vi "test data analysis.vi"() -> ()   [LabVIEW 2013]
uses:
  <vilib>/Utility/file.llb/Read From Spreadsheet File (string).vi
panel:
  out "Pick up Balance  2":cluster{dbl[], dbl[]}(graph)
  in  "탭 컨트롤":enum32{"페이지 1", "페이지 2"}(tab)
  out "Bonding Balance":cluster{dbl[], dbl[]}(graph)
  out "Pick up Balance":cluster{dbl[], dbl[]}(graph)
  out "숫자형":i32
  out "Balance all":cluster{dbl[], dbl[]}(graph)
  in  "balance y":i32
  in  "balance x":i32
  in  "time index 2":i32
  out "temp 그래프 4":dbl[](graph)
  out "temp 그래프 3":dbl[](graph)
  in  "vacuum index":i32
  out "temp 그래프 2":dbl[](graph)
  in  "temp index":i32
  in  "force index":i32
  out "웨이브폼 그래프":dbl[](graph)
  in  "file path":path caption="Data file path"
  out "Data Table":string[][](table)
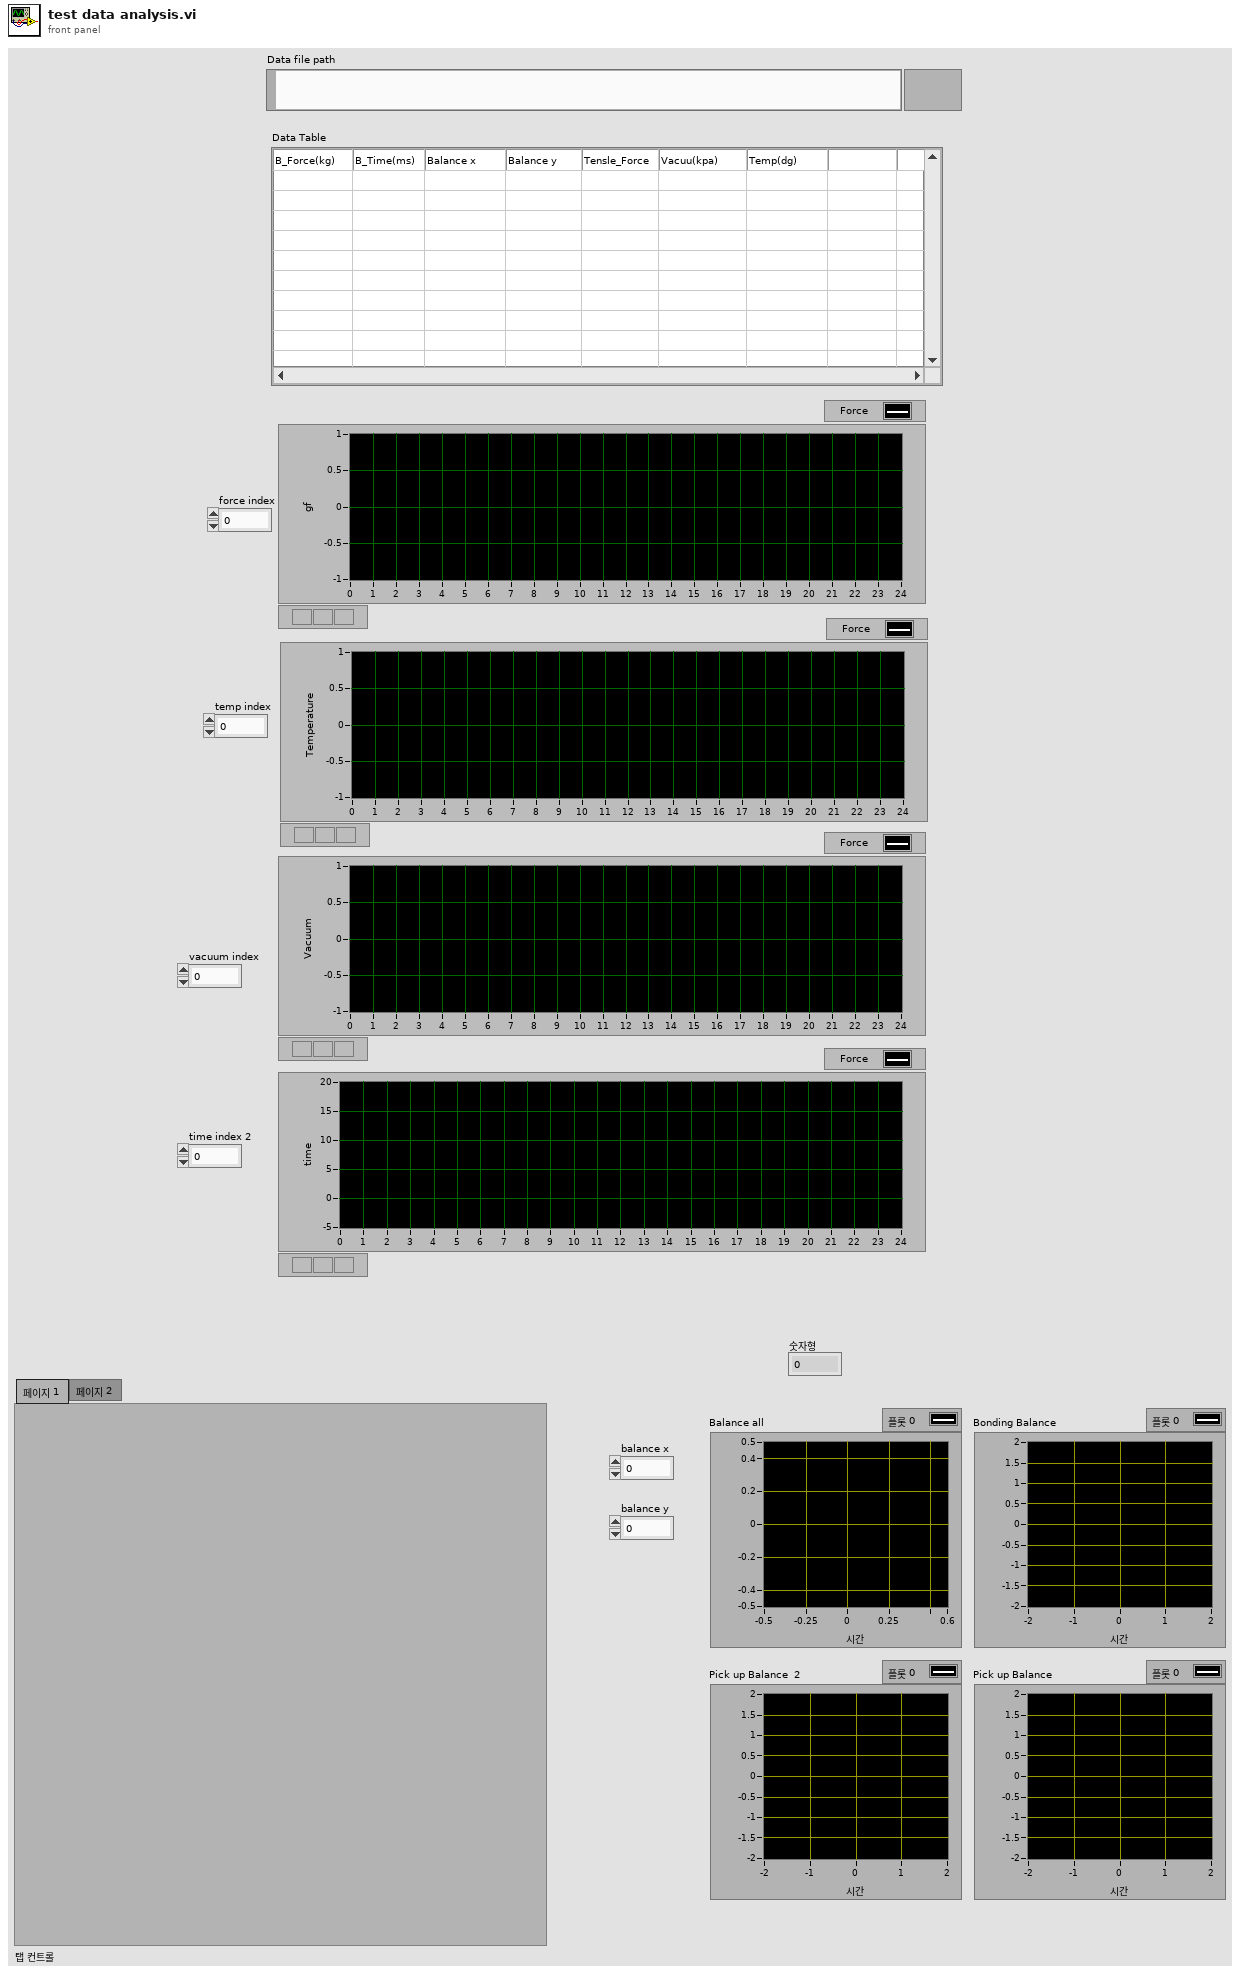
[diagram p1: front panel]
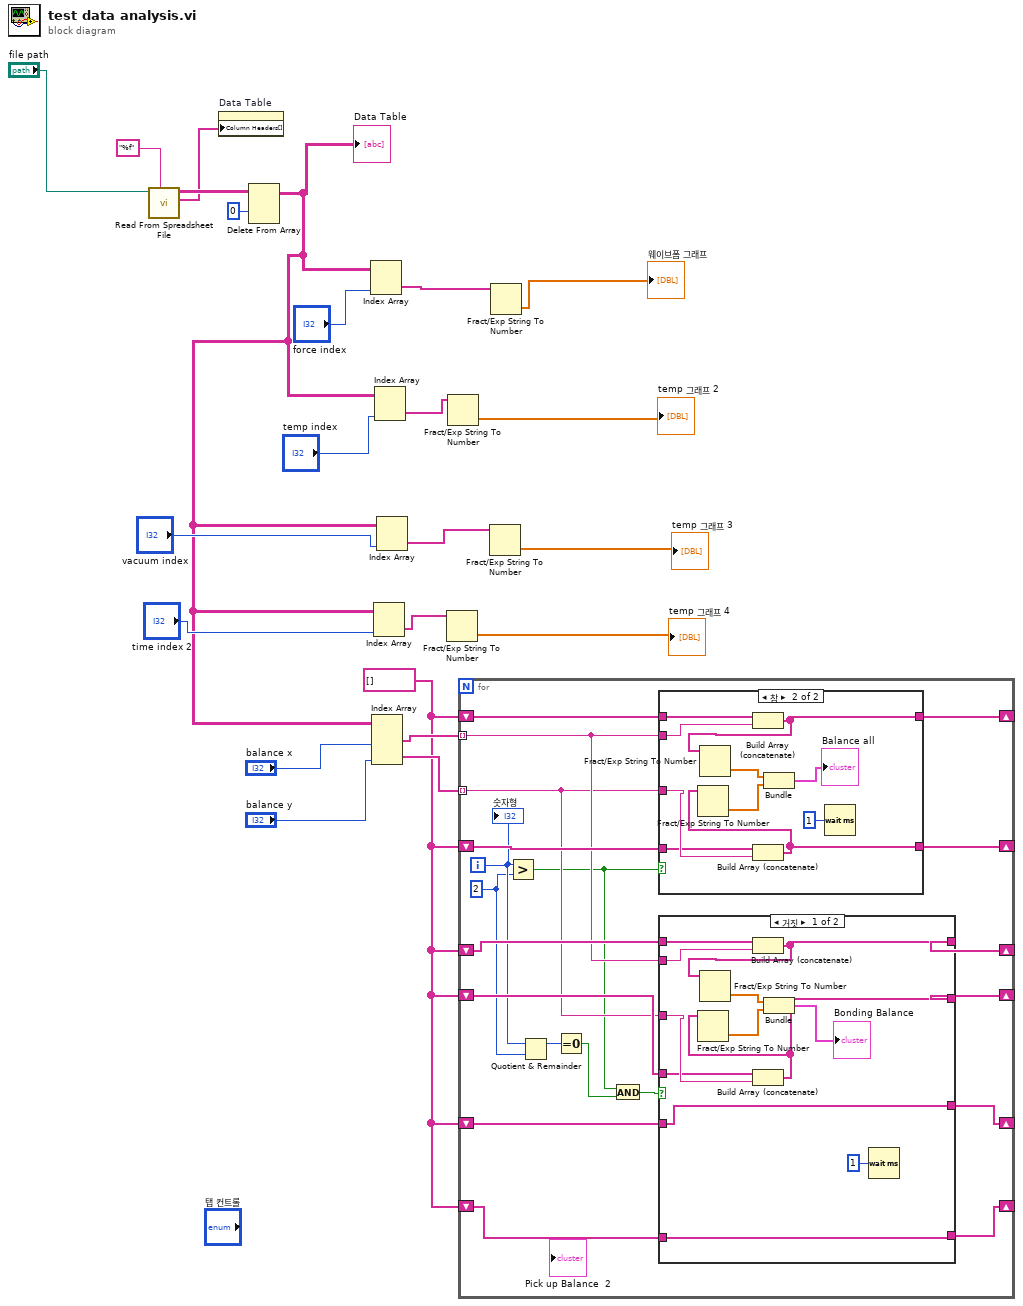
[diagram p0: block diagram]
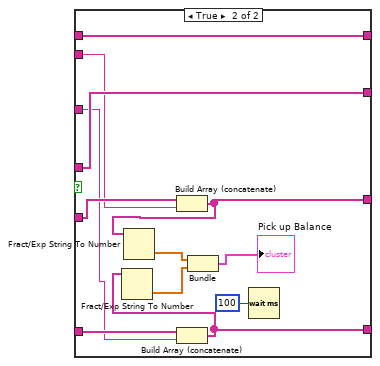
[diagram p2: hidden frame]
diagram:
  w1 = string[] []
  n1 = call-poly <vilib>:"Read From Spreadsheet File.vi"("format (%s)"="%f", "file path (dialog if empty)"="file path") -> ("first row"=w20:string[], "all rows"=w22:string[][])  [unwired: 5 in, 3 out]
  n2 = property on="Data Table" class="Tbl (엄격한)"("Column Headers[]"=w20) -> ()  [unwired: 2 in, 2 out]
  n3 = Delete From Array(array=w22, index (row)=0 ("인덱스 (행)")) -> (array with subset deleted=w5:string[][])  [unwired: 2 in, 1 out]
  "Data Table" <- w5
  n4 = Index Array(array=w5, index (col)="force index") -> (element=w18:string[])  [unwired: 1 in]
  n5 = Index Array(array=w5, index (col) #1="balance x", index (col) #2="balance y") -> (element #1=w6:string[], element #2=w2:string[])  [unwired: 2 in]
  n6 = Index Array(array=w5, index (col)="time index 2") -> (element=w8:string[])  [unwired: 1 in]
  n7 = Index Array(array=w5, index (col)="temp index") -> (element=w14:string[])  [unwired: 1 in]
  n8 = Index Array(array=w5, index (col)="vacuum index") -> (element=w12:string[])  [unwired: 1 in]
  n9 = Fract/Exp String To Number(string=w8) -> (number=→"temp 그래프 4":dbl[])  [unwired: 3 in, 1 out]
  n10 = Fract/Exp String To Number(string=w14) -> (number=→"temp 그래프 2":dbl[])  [unwired: 3 in, 1 out]
  n11 = for {
    tunnel: w6 -> [w37] mode=indexing
    tunnel: w2 -> [w36] mode=indexing
    shift-right: [w40] -> _
    shift-left: w1 -> [w41]
    shift-right: [w42] -> _
    shift-left: w1 -> [w43]
    shift-right: [w29] -> _
    shift-left: w1 -> [w39]
    shift-right: [w26] -> _
    shift-left: w1 -> [w38]
    shift-right: [w24] -> _
    shift-left: w1 -> [w28]
    shift-right: [w25] -> _
    shift-left: w1 -> [w27]
    i -> [w35]
    w34 = 2 ("y")
    n12 = Greater?(x=w35, y=w34) -> (0:w32:bool)
    n13 = Quotient & Remainder(x=w35, y=w34) -> (x-y*floor(x/y)=w33:i32)  [unwired: 1 out]
    n14 = Equal To 0?(x=w33) -> (x = 0?=w31:bool)
    n15 = And(x=w32, y=w31) -> (x .and. y?=w30:bool)
    n16 = case shown="참" w32 {
      tunnel: w43 -> [w69 w76]
      tunnel: w37 -> [_ w75]
      tunnel: [w69 w74] -> w42
      tunnel: w36 -> [_ w73]
      tunnel: w41 -> [w68 w72]
      tunnel: [w68 w71] -> w40
      frame False {
      }
      frame True {
        n17 = Build Array (concatenate)(w76, w75) -> (w74:string[])
        n18 = Fract/Exp String To Number(string=w74) -> (number=w78:dbl[])  [unwired: 3 in, 1 out]
        n19 = Build Array (concatenate)(w72, w73) -> (w71:string[])
        n20 = Fract/Exp String To Number(string=w71) -> (number=w79:dbl[])  [unwired: 3 in, 1 out]
        n21 = Bundle(w78, w79) -> (→"Balance all":cluster{dbl[], dbl[]})  [unwired: 1 in]
        n22 = Wait (ms)(milliseconds to wait=u32 1 ("대기 시간(ms)")) -> ()  [unwired: 1 out]
      }
    }
    n23 = case shown="거짓" w30 {
      tunnel: w39 -> [w52 w67]
      tunnel: w37 -> [w51 w57]
      tunnel: [w50 w67] -> w29
      tunnel: w36 -> [w49 w56]
      tunnel: w38 -> [w48 w66]
      tunnel: [w47 w66] -> w26
      tunnel: w28 -> [w45 w61]
      tunnel: w27 -> [w44 w60]
      tunnel: [w44 w59] -> w25
      tunnel: [w45 w58] -> w24
      frame False {
        n24 = Build Array (concatenate)(w52, w51) -> (w50:string[])
        n25 = Fract/Exp String To Number(string=w50) -> (number=w54:dbl[])  [unwired: 3 in, 1 out]
        n26 = Build Array (concatenate)(w48, w49) -> (w47:string[])
        n27 = Fract/Exp String To Number(string=w47) -> (number=w55:dbl[])  [unwired: 3 in, 1 out]
        n28 = Bundle(w54, w55) -> (→"Bonding Balance":cluster{dbl[], dbl[]})  [unwired: 1 in]
        n29 = Wait (ms)(milliseconds to wait=u32 1 ("대기 시간(ms)")) -> ()  [unwired: 1 out]
      }
      frame True {
        n30 = Build Array (concatenate)(w61, w57) -> (w58:string[])
        n31 = Fract/Exp String To Number(string=w58) -> (number=w64:dbl[])  [unwired: 3 in, 1 out]
        n32 = Build Array (concatenate)(w60, w56) -> (w59:string[])
        n33 = Fract/Exp String To Number(string=w59) -> (number=w63:dbl[])  [unwired: 3 in, 1 out]
        n34 = Bundle(w64, w63) -> (→"Pick up Balance":cluster{dbl[], dbl[]})  [unwired: 1 in]
        n35 = Wait (ms)(milliseconds to wait=u32 100 ("대기 시간(ms)")) -> ()  [unwired: 1 out]
      }
    }
    "숫자형" <- w35
  }
  n36 = Fract/Exp String To Number(string=w12) -> (number=→"temp 그래프 3":dbl[])  [unwired: 3 in, 1 out]
  n37 = Fract/Exp String To Number(string=w18) -> (number=→"웨이브폼 그래프":dbl[])  [unwired: 3 in, 1 out]
